vi "Enqueue FirstHandshake Connection.vi"(8 "Error In":errorcluster, 10 "Barcode":string, 11 "Name":string) -> (0 "Error Out":errorcluster, 2 "Result":string)   [LabVIEW 2019, in "TCP2Foxconn.lvlib"]
uses:
  TCP2Foxconn.lvlib
  Queue/Queue.lvlib
  Data Error Notifier/Data and Error Notifier.lvlib
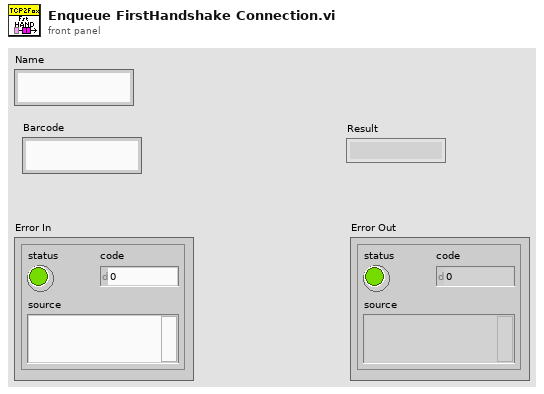
[diagram p1: front panel]
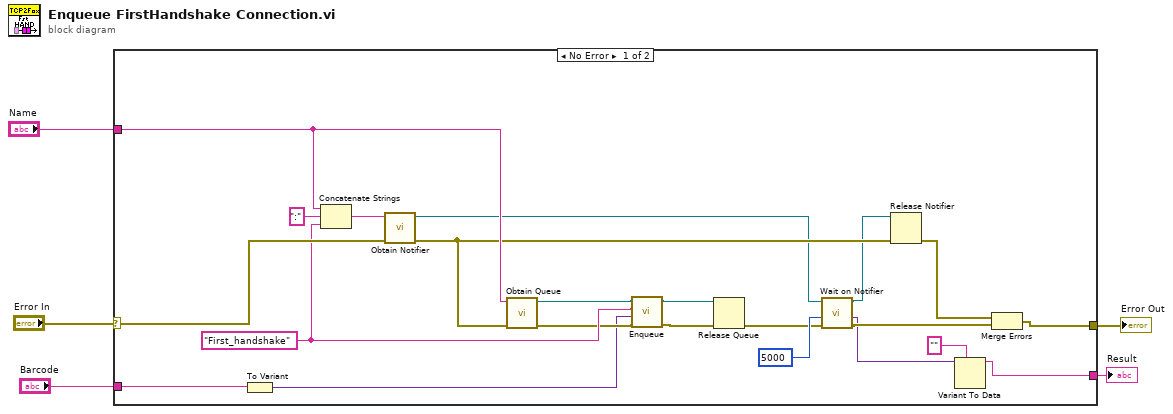
[diagram p0: block diagram]
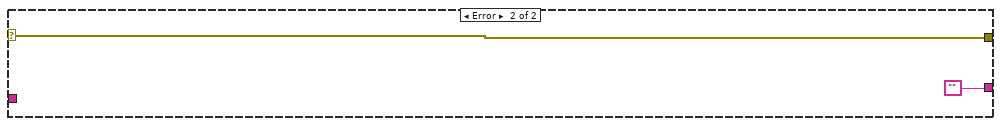
[diagram p2: hidden frame]
diagram:
  n1 = case shown="No Error" "Error In" {
    selector: "Error In" -> [w22 w29]
    tunnel: [w24 w29] -> w4
    tunnel: "Name" -> [w27 _]
    tunnel: [w9 ""] -> w1
    tunnel: "Barcode" -> [w8 _]
    frame No Error {
      w19 = "First_handshake" ("Message")
      n2 = To Variant(anything=w8) -> (Variant=w7:variant)
      n3 = Concatenate Strings(w27, ":" ("string"), w19) -> (w23:string)
      n4 = call "Obtain Notifier.vi"("Error In"=w22, "Name"=w23) -> ("Error Out"=w21:errorcluster, "notifier out"=w15:refnum<notifier>)  [unwired: 8 in]
      n5 = call "Obtain Queue.vi"("Error In"=w21, "Name"=w27) -> ("Error Out"=w18:errorcluster, "queue out"=w20:refnum<queue>)  [unwired: 8 in]
      n6 = call "Enqueue.vi"("Error In"=w18, "Data"=w7, "Message"=w19, "queue in"=w20) -> ("Error Out"=w16:errorcluster, "queue out"=w17:refnum<queue>)  [unwired: 6 in]
      n7 = Release Queue(queue=w17, error in (no error)=w16) -> (error out=w13:errorcluster)  [unwired: 1 in, 2 out]
      n8 = call "Wait on Notifier.vi"("Error In"=w13, "timeout in ms (-1)"=5000, "notifier in"=w15) -> ("Error Out"=w11:errorcluster, "Data"=w10:variant, "notifier out"=w12:refnum<notifier>)  [unwired: 6 in]
      n9 = Release Notifier(notifier=w12, error in (no error)=w21) -> (error out=w25:errorcluster)  [unwired: 1 in, 2 out]
      n10 = Variant To Data(type="", Variant=w10) -> (data=w9:string)  [unwired: 1 in, 1 out]
      n11 = Merge Errors(w25, w11) -> (w24:errorcluster)
    }
    frame Error {
    }
  }
  "Error Out" <- w4
  "Result" <- w1
